vi "Get FOV control info.vi"(8 "error in (no error)":errorcluster) -> (0 "error out":errorcluster, 1 "Number of different FOVs":i32, 2 "FOV values cluster":T1, 3 "FOV selection index":i32)   [LabVIEW 2013]
uses:
  Typedefs/FOV values cluster.ctl
  <vilib>/Utility/miscctls.llb/LVStringsAndValuesArrayTypeDef_SGL.ctl
  Global Variables/gl_UI Ctrl Refs.vi
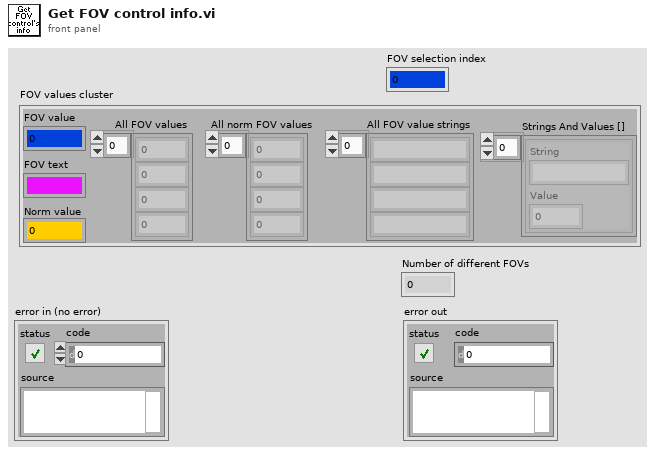
[diagram p1: front panel]
types:
  T1 = typedef "FOV values cluster.ctl" = cluster{"Norm value":sgl, "FOV text":string, "FOV value":i32, "All FOV values":i32[], "All norm FOV values":sgl[], "All FOV value strings":string[], "Strings And Values []":T2}
  T2 = typedef "LVStringsAndValuesArrayTypeDef_SGL.ctl" = cluster{"String":string, "Value":sgl}[]
  T3 = typedef "UI ctrl refs cluster.ctl" = cluster{"Top level VI path":path, "Top level VI ref":refnum<vi>, "User menu ref":refnum<k9>, "Sub Panel control":refnum<vi>, "Imaging Param Tab":refnum<vi>, "Occurrence-Start drivers":refnum<k4>, "Occurrence-Speed logging initialised":refnum<k4>, "Occurrence-XYZ stage initialised":refnum<k4>, "Exit button":refnum<vi>, "Status ind":refnum<vi>, "Return to Origin":refnum<vi>, "Speed Logging":refnum<vi>, "Time Lapse":refnum<vi>, "Live Imaging":refnum<vi>, "AOL Z Stack":refnum<vi>, "Motor Z Stack":refnum<vi>, "Funct Acq button":refnum<vi>, "Hard Shutter":refnum<vi>, "Virtual Shutter":refnum<vi>, "Laser Power":refnum<vi>, "AOL Mode":refnum<vi>, "Frame Size":refnum<vi>, "Field of View":refnum<vi>, "Dwell Time":refnum<vi>, "Zoom":refnum<vi>, "AOL Z":refnum<vi>, "Objective":refnum<vi>, "Axis":refnum<vi>, "Paths & Names":refnum<vi>, "Experiment folder path (ind.)":refnum<vi>, "Last State (Ind.)":refnum<vi>, "Laser wavelength ind (nm)":refnum<vi>, "Averages":refnum<vi>, "Angle (degrees)":refnum<vi>, "X centre":refnum<vi>, "Y centre":refnum<vi>, "Plane Mode":refnum<vi>, "# Planes":refnum<vi>, "Z Start":refnum<vi>, "Z Stop":refnum<vi>, "Z Step":refnum<vi>, "PMT 1":refnum<vi>, "PMT 2":refnum<vi>, "Stage XYZ Position":refnum<vi>, "Pockels@Z Start":refnum<vi>, "Pockels@Z Stop":refnum<vi>, "Obtain Z Start":refnum<vi>, "Obtain Z Stop":refnum<vi>, "Live stim.trig.period":refnum<vi>, "Live stim.trig.enable":refnum<vi>, "Funct. Acq. Pockels Modulation":refnum<vi>, "Enable Video Recording":refnum<vi>, "Video Record-Live Imaging":refnum<vi>, "Video Record-Funct acq":refnum<vi>, "AOL Z-stack Chirps Ready (ind)":refnum<vi>, "Center freq ind (nm)":refnum<vi>, "Logging queue (ind)":refnum<vi>, "Back aperture power (ind.)":refnum<vi>, "Power after objective (ind.)":refnum<vi>, "Switch user":refnum<vi>}
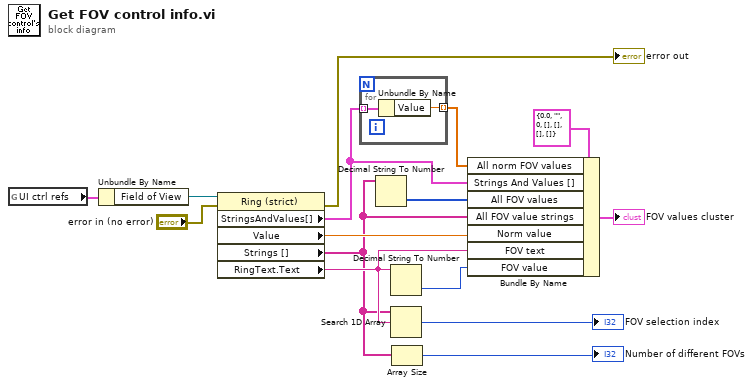
[diagram p0: block diagram]
diagram:
  n1 = global read "gl_UI Ctrl Refs.vi" "UI ctrl refs"() -> (w12:T3)
  n2 = Unbundle By Name(w12) -> ("Field of View"=w11:refnum<vi>)
  n3 = property on="Property Node" class="Ring (strict)"(reference=w11, error in="error in (no error)") -> (error out=→"error out":errorcluster, "StringsAndValues[]"=w2:T2, "Value"=w5:sgl, "Strings []"=w4:string[], "RingText.Text"=w7:string)  [unwired: 1 out]
  n4 = for {
    tunnel: w2 -> [w17] mode=indexing
    tunnel: [w16] -> w1 mode=indexing
    n5 = Unbundle By Name(w17) -> ("Value"=w16:sgl)
  }
  n6 = Decimal String To Number(string=w4) -> (number=w9:i32[])  [unwired: 2 in, 1 out]
  n7 = Decimal String To Number(string=w7) -> (number=w8:i32)  [unwired: 2 in, 1 out]
  n8 = Search 1D Array(1D array=w4, element=w7) -> (index of element=→"FOV selection index":i32)  [unwired: 1 in]
  n9 = Array Size(array=w4) -> (size(s)=→"Number of different FOVs":i32)
  n10 = Bundle By Name(cluster=T1 {"Norm value"=0.0, "FOV text"="", "FOV value"=0, "All FOV values"=[], "All norm FOV values"=[], "All FOV value strings"=[], "Strings And Values []"=[]} ("FOV values cluster"), "All norm FOV values"=w1, "Strings And Values []"=w2, "All FOV values"=w9, "All FOV value strings"=w4, "Norm value"=w5, "FOV text"=w7, "FOV value"=w8) -> (→"FOV values cluster":T1)
